vi "SwitchFinder.vi"(10 "All Lines in":T1) -> (2 "All Lines out":T1)   [LabVIEW 2014]
uses:
  Libraries/Map Data Folder/All-Lines.ctl
  Libraries/Map Data Folder/LineCluster.ctl
  Libraries/Map Data Folder/LineConnection.ctl
  Libraries/Map Data Folder/Map Data.lvlib
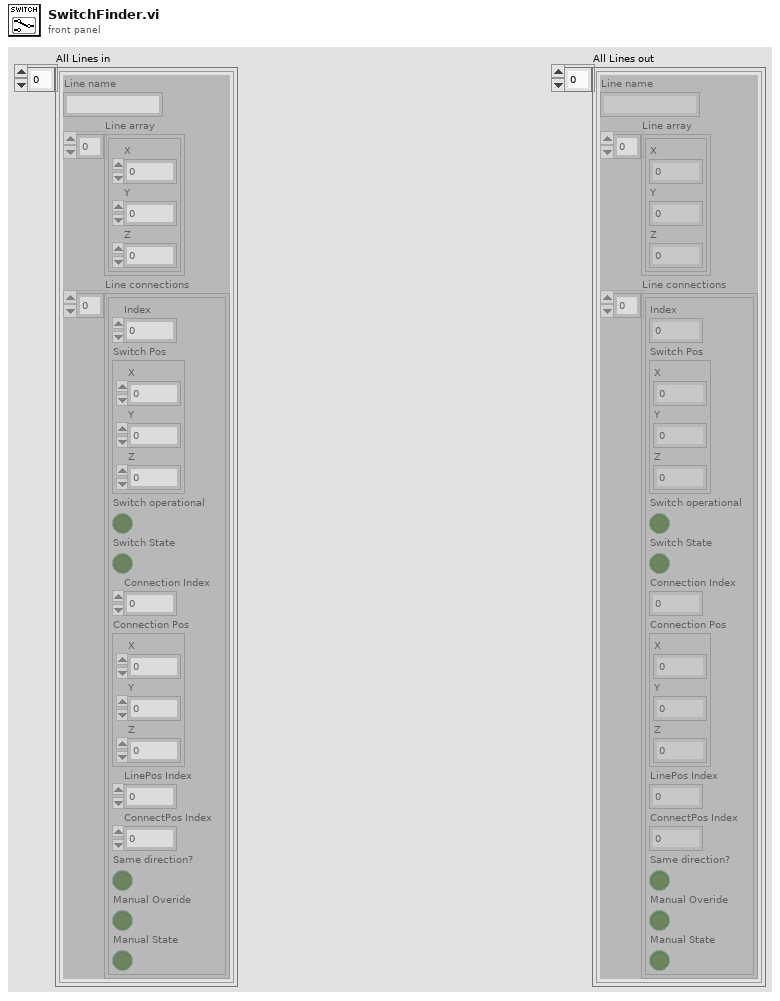
[diagram p1: front panel]
types:
  T1 = typedef "Map Data.lvlib/All-Lines.ctl" = T2[]
  T2 = typedef "Map Data.lvlib/LineCluster.ctl" = cluster{"Line name":string, "Line array":cluster{"X":dbl, "Y":dbl, "Z":dbl}[], "Line connections":T3[]}
  T3 = typedef "LineConnection.ctl" = cluster{"Index":i32, "Switch Pos":cluster{"X":dbl, "Y":dbl, "Z":dbl}, "Switch operational":bool, "Switch State":bool, "Connection Index":i32, "Connection Pos":cluster{"X":dbl, "Y":dbl, "Z":dbl}, "LinePos Index":i32, "ConnectPos Index":i32, "Same direction?":bool, "Manual Overide":bool, "Manual State":bool}
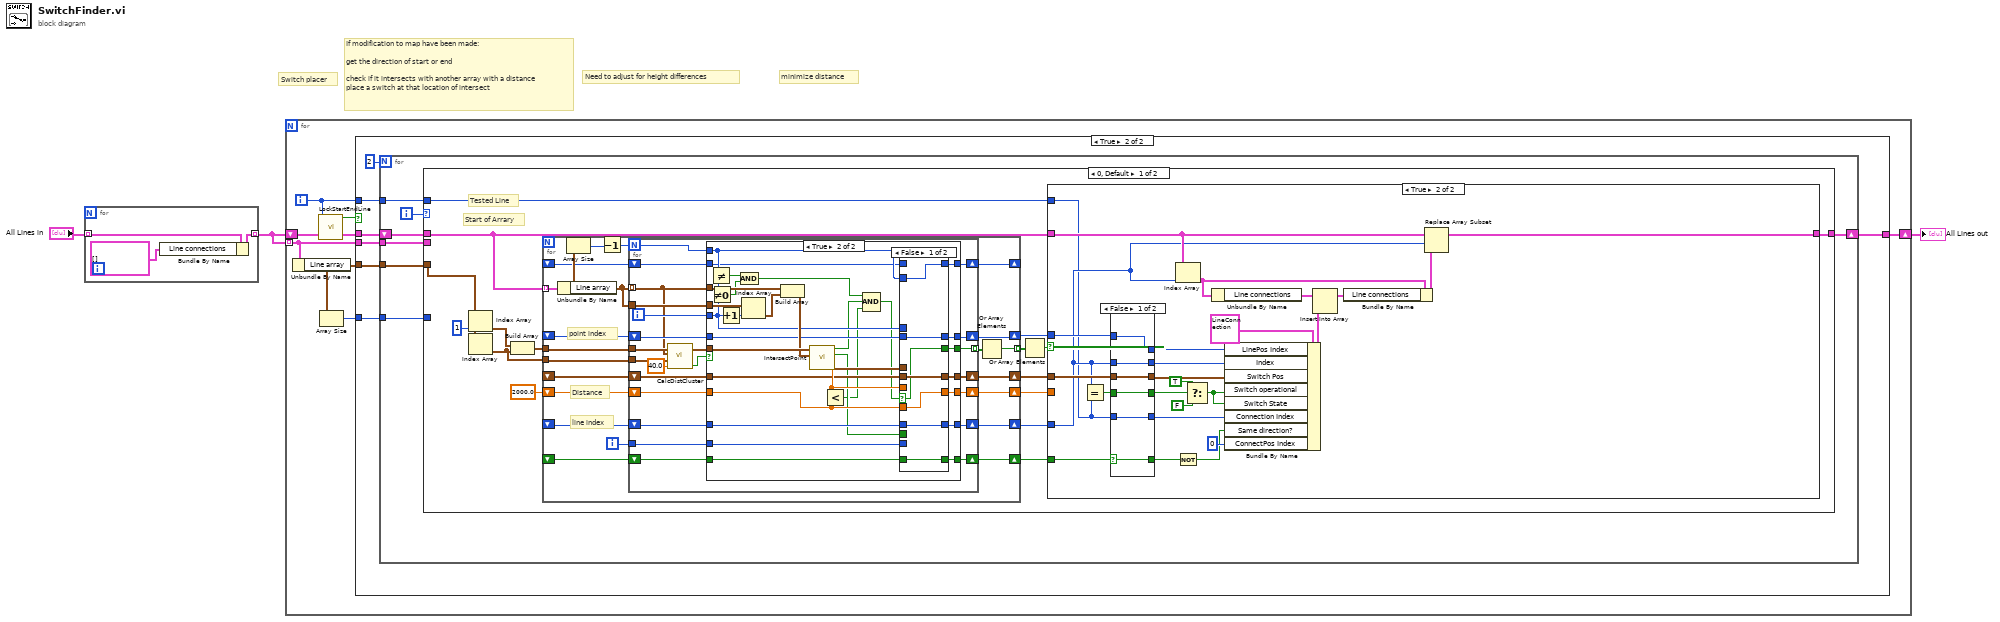
[diagram p0: block diagram]
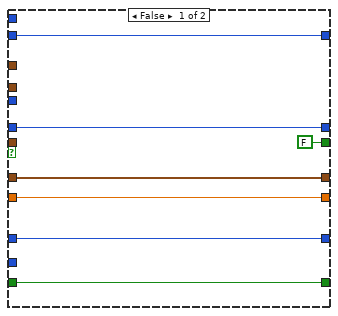
[diagram p5: hidden frame]
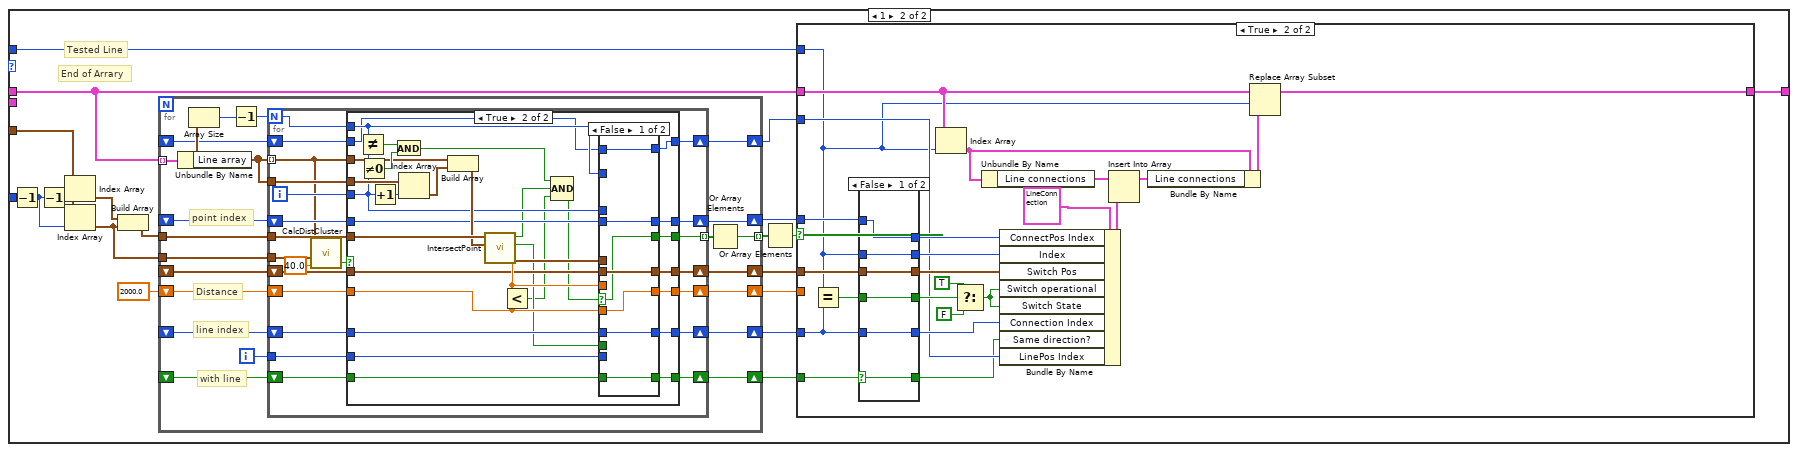
[diagram p7: hidden frame]
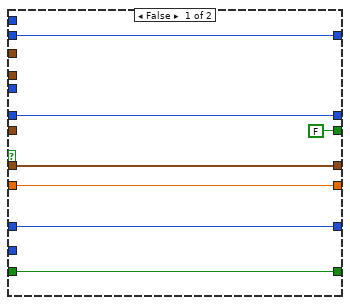
[diagram p10: hidden frame]
diagram:
  # "minimize distance"
  # "Need to adjust for height differences"
  # "If modification to map have been made:\n\nget the direction of start or end\n\ncheck if it intersects with another array with a distance\nplace a switch at that location of intersect"
  # "Switch placer"
  n1 = for {
    tunnel: [w5] -> w2 mode=indexing
    tunnel: "All Lines in" -> [w6] mode=indexing
    n2 = Bundle By Name(cluster=w6, "Line connections"=T3[] []) -> (w5:T2)
  }
  n3 = for {
    tunnel: w2 -> [w10] mode=indexing
    shift-right: [w7] -> w3
    shift-left: w2 -> [w9]
    i -> [w8]
    n4 = Unbundle By Name(w10) -> ("Line array"=w12:cluster{"X":dbl, "Y":dbl, "Z":dbl}[])
    n5 = call "LockStartEndLine.vi"("index"=w8, "All Lines"=w9) -> ("Not Locked?"=w11:bool)  [unwired: 9 in]
    n6 = Array Size(array=w12) -> (size(s)=w13:i32)
    n7 = case shown="True" w11 {
      tunnel: w13 -> [_ w21]
      tunnel: w12 -> [_ w20]
      tunnel: w10 -> [_ w16]
      tunnel: w9 -> [w14 w18]
      tunnel: w8 -> [_ w17]
      tunnel: [w14 w15] -> w7
      frame False {
      }
      frame True {
        n8 = for {
          N: 2 -> [_]
          tunnel: w21 -> [w28]
          tunnel: w20 -> [w27]
          shift-right: [w24] -> w15
          shift-left: w18 -> [w25]
          tunnel: w17 -> [w23]
          tunnel: w16 -> [w22]
          i -> [w26]
          n9 = case shown="0, Default" w26 {
            tunnel: w28 -> [_ w183]
            tunnel: w27 -> [w42 w194]
            tunnel: w25 -> [w37 w190]
            tunnel: [w38 w191] -> w24
            tunnel: w23 -> [w36 w189]
            tunnel: w22 -> [_ _]
            frame 0, Default {
              # "Tested Line"
              # "Start of Arrary"
              n10 = Index Array(array=w42, index=1) -> (element=w44:cluster{"X":dbl, "Y":dbl, "Z":dbl})
              n11 = Index Array(array=w42) -> (element=w30:cluster{"X":dbl, "Y":dbl, "Z":dbl})  [unwired: 1 in]
              n12 = Build Array(w44, w30) -> (w43:cluster{"X":dbl, "Y":dbl, "Z":dbl}[])
              n13 = for {
                tunnel: w43 -> [w103]
                tunnel: w37 -> [w102] mode=indexing
                shift-right: [w99] -> w32
                shift-left: 2000.0 ("Distance") -> [w98]
                shift-right: [w96] -> w34
                shift-left: _ -> [w95]
                shift-right: [w92] -> w31
                shift-left: _ -> [w93]
                tunnel: [w90] -> w40 mode=indexing
                shift-right: [w89] -> w33
                shift-left: _ -> [w88]
                tunnel: w30 -> [w87]
                shift-right: [w86] -> w29
                shift-left: _ -> [w85]
                shift-right: [w84] -> _
                shift-left: _ -> [w83]
                i -> [w91]
                # "Distance"
                # "line index"
                # "point index"
                n14 = Unbundle By Name(w102) -> ("Line array"=w101:cluster{"X":dbl, "Y":dbl, "Z":dbl}[])
                n15 = Array Size(array=w101) -> (size(s)=w94:i32)
                n16 = Decrement(x=w94) -> (x-1=w100:i32)
                n17 = for {
                  N: w100 -> [w117]
                  tunnel: w103 -> [w125]
                  tunnel: w101 -> [w109] mode=indexing
                  tunnel: w101 -> [w124]
                  tunnel: [w120] -> w97 mode=indexing
                  shift-right: [w122] -> w99
                  shift-left: w98 -> [w123]
                  shift-right: [w121] -> w96
                  shift-left: w95 -> [w119]
                  tunnel: w91 -> [w115]
                  shift-right: [w116] -> w92
                  shift-left: w93 -> [w114]
                  shift-right: [w113] -> w89
                  shift-left: w88 -> [w112]
                  tunnel: w87 -> [w108]
                  shift-right: [w107] -> w86
                  shift-left: w85 -> [w106]
                  shift-right: [w105] -> w84
                  shift-left: w83 -> [w104]
                  i -> [w118]
                  n18 = call "CalcDistCluster.vi"("Less than"=40.0, "element 2"=w108, "element"=w109) -> ("Less than?"=w110:bool)  [unwired: 7 in, 1 out]
                  n19 = case shown="True" w110 {
                    tunnel: w125 -> [_ w163]
                    tunnel: w124 -> [_ w162]
                    tunnel: w109 -> [_ w160]
                    tunnel: w123 -> [w129 w157]
                    tunnel: [w129 w155] -> w122
                    tunnel: [w132 w154] -> w121
                    tunnel: [FALSE w153] -> w120
                    tunnel: w119 -> [w132 w152]
                    tunnel: w118 -> [_ w151]
                    tunnel: w117 -> [_ w139]
                    tunnel: [w128 w148] -> w116
                    tunnel: w115 -> [_ w147]
                    tunnel: w114 -> [w128 w146]
                    tunnel: [w130 w144] -> w113
                    tunnel: w112 -> [w130 w143]
                    tunnel: [w127 w141] -> w107
                    tunnel: w106 -> [w127 w140]
                    tunnel: [w126 w138] -> w105
                    tunnel: w104 -> [w126 w137]
                    frame False {
                    }
                    frame True {
                      n20 = Not Equal?(x=w139, y=w151) -> (x != y?=w150:bool)
                      n21 = Not Equal To 0?(x=w151) -> (x != 0?=w149:bool)
                      n22 = Increment(x=w151) -> (x+1=w161:i32)
                      n23 = And(x=w150, y=w149) -> (x .and. y?=w136:bool)
                      n24 = Index Array(array=w162, index=w161) -> (element=w159:cluster{"X":dbl, "Y":dbl, "Z":dbl})
                      n25 = Build Array(w160, w159) -> (w158:cluster{"X":dbl, "Y":dbl, "Z":dbl}[])
                      n26 = call "IntersectPoint.vi"("Against Array"=w158, "Test Array"=w163) -> ("Intersect Point"=w145:cluster{"X":dbl, "Y":dbl, "Z":dbl}, "Distance"=w156:dbl, "With Line?"=w142:bool, "Check"=w135:bool)  [unwired: 6 in]
                      n27 = Less?(x=w156, y=w157) -> (x < y?=w134:bool)
                      n28 = Compound Arithmetic op=AND(w136, w135, w134) -> (w133:bool)
                      n29 = case shown="False" w133 {
                        selector: w133 -> [w164 w171]
                        tunnel: w157 -> [w170 _]
                        tunnel: w156 -> [_ w177]
                        tunnel: [w170 w177] -> w155
                        tunnel: w152 -> [w169 _]
                        tunnel: [w169 w176] -> w154
                        tunnel: [w164 w171] -> w153
                        tunnel: w151 -> [_ w176]
                        tunnel: [w168 w175] -> w148
                        tunnel: w147 -> [_ w175]
                        tunnel: w146 -> [w168 _]
                        tunnel: w145 -> [_ w174]
                        tunnel: [w167 w174] -> w144
                        tunnel: w143 -> [w167 _]
                        tunnel: w142 -> [_ w173]
                        tunnel: [w166 w173] -> w141
                        tunnel: w140 -> [w166 _]
                        tunnel: w139 -> [w165 _]
                        tunnel: [w165 w172] -> w138
                        tunnel: w137 -> [_ w172]
                        frame False {
                        }
                        frame True {
                        }
                      }
                    }
                  }
                }
                n30 = Or Array Elements(Boolean array=w97) -> (logical OR=w90:bool)
              }
              n31 = Or Array Elements(Boolean array=w40) -> (logical OR=w35:bool)
              n32 = case shown="True" w35 {
                tunnel: [w45 w50] -> w38
                tunnel: w37 -> [w45 w66]
                tunnel: w36 -> [_ w48]
                tunnel: w34 -> [_ w56]
                tunnel: w33 -> [_ w64]
                tunnel: w32 -> [_ _]
                tunnel: w31 -> [_ w49]
                tunnel: w29 -> [_ w65]
                frame False {
                }
                frame True {
                  n33 = Equal?(x=w49, y=w48) -> (x = y?=w58:bool)
                  n34 = case shown="False" w65 {
                    selector: w65 -> [w71 w78]
                    tunnel: w48 -> [w75 w82]
                    tunnel: [w75 w82] -> w62
                    tunnel: [w76 w81] -> w51
                    tunnel: w64 -> [w76 w81]
                    tunnel: w49 -> [w74 w77]
                    tunnel: [w74 w77] -> w63
                    tunnel: w58 -> [w73 w80]
                    tunnel: [w73 w80] -> w57
                    tunnel: w56 -> [w72 w79]
                    tunnel: [w72 w79] -> w53
                    tunnel: [w71 w78] -> w54
                    frame False {
                    }
                    frame True {
                    }
                  }
                  n35 = Index Array(array=w66, index=w49) -> (element=w70:T2)
                  n36 = Not(x=w54) -> (.not. x?=w47:bool)
                  n37 = Select(t=TRUE ("Switch operational"), s=w57, f=FALSE ("Switch operational")) -> (s? t:f=w61:bool)
                  n38 = Unbundle By Name(w70) -> ("Line connections"=w67:T3[])
                  n39 = Bundle By Name(cluster=T3 {"Index"=0, "Switch Pos"={"X"=0.0, "Y"=0.0, "Z"=0.0}, "Switch operational"=FALSE, "Switch State"=FALSE, "Connection Index"=0, "Connection Pos"={"X"=0.0, "Y"=0.0, "Z"=0.0}, "LinePos Index"=0, "ConnectPos Index"=0, "Same direction?"=FALSE, "Manual Overide"=FALSE, "Manual State"=FALSE}, "LinePos Index"=w53, "Index"=w63, "Switch Pos"=w51, "Switch operational"=w61, "Switch State"=w61, "Connection Index"=w62, "Same direction?"=w47, "ConnectPos Index"=0) -> (w55:T3)
                  n40 = Insert Into Array(array=w67, new element=w55) -> (w69:T3[])  [unwired: 1 in]
                  n41 = Bundle By Name(cluster=w70, "Line connections"=w69) -> (w68:T2)
                  n42 = Replace Array Subset(array=w66, new element=w68, index=w49) -> (w50:T2[])
                }
              }
            }
            frame 1 {
              # "Tested Line"
              # "End of Arrary"
              n43 = Decrement(x=w183) -> (x-1=w182:i32)
              n44 = Decrement(x=w182) -> (x-1=w181:i32)
              n45 = Index Array(array=w194, index=w181) -> (element=w196:cluster{"X":dbl, "Y":dbl, "Z":dbl})
              n46 = Index Array(array=w194, index=w182) -> (element=w180:cluster{"X":dbl, "Y":dbl, "Z":dbl})
              n47 = Build Array(w196, w180) -> (w195:cluster{"X":dbl, "Y":dbl, "Z":dbl}[])
              n48 = for {
                tunnel: w195 -> [w254]
                tunnel: w190 -> [w253] mode=indexing
                shift-right: [w250] -> w185
                shift-left: 2000.0 ("Distance") -> [w249]
                shift-right: [w247] -> w187
                shift-left: _ -> [w246]
                shift-right: [w243] -> w184
                shift-left: _ -> [w244]
                tunnel: [w241] -> w192 mode=indexing
                shift-right: [w240] -> w186
                shift-left: _ -> [w239]
                tunnel: w180 -> [w238]
                shift-right: [w237] -> w179
                shift-left: _ -> [w236]
                shift-right: [w235] -> w178
                shift-left: _ -> [w234]
                i -> [w242]
                # "with line"
                # "Distance"
                # "line index"
                # "point index"
                n49 = Unbundle By Name(w253) -> ("Line array"=w252:cluster{"X":dbl, "Y":dbl, "Z":dbl}[])
                n50 = Array Size(array=w252) -> (size(s)=w245:i32)
                n51 = Decrement(x=w245) -> (x-1=w251:i32)
                n52 = for {
                  N: w251 -> [w257]
                  tunnel: w254 -> [w276]
                  tunnel: w252 -> [w263] mode=indexing
                  tunnel: w252 -> [w275]
                  tunnel: [w271] -> w248 mode=indexing
                  shift-right: [w273] -> w250
                  shift-left: w249 -> [w274]
                  shift-right: [w272] -> w247
                  shift-left: w246 -> [w270]
                  tunnel: w242 -> [w267]
                  shift-right: [w268] -> w243
                  shift-left: w244 -> [w266]
                  shift-right: [w265] -> w240
                  shift-left: w239 -> [w264]
                  tunnel: w238 -> [w262]
                  shift-right: [w259] -> w237
                  shift-left: w236 -> [w258]
                  shift-right: [w256] -> w235
                  shift-left: w234 -> [w255]
                  i -> [w269]
                  n53 = call "CalcDistCluster.vi"("Less than"=40.0, "element 2"=w262, "element"=w263) -> ("Less than?"=w260:bool)  [unwired: 7 in, 1 out]
                  n54 = case shown="True" w260 {
                    tunnel: w276 -> [_ w314]
                    tunnel: w275 -> [_ w313]
                    tunnel: w274 -> [w280 w309]
                    tunnel: [w280 w307] -> w273
                    tunnel: [w283 w306] -> w272
                    tunnel: [FALSE w305] -> w271
                    tunnel: w270 -> [w283 w304]
                    tunnel: w269 -> [_ w303]
                    tunnel: [w281 w300] -> w268
                    tunnel: w267 -> [_ w299]
                    tunnel: w266 -> [w281 w298]
                    tunnel: [w282 w296] -> w265
                    tunnel: w264 -> [w282 w295]
                    tunnel: w263 -> [_ w294]
                    tunnel: [w278 w292] -> w259
                    tunnel: w258 -> [w278 w291]
                    tunnel: w257 -> [_ w290]
                    tunnel: [w277 w288] -> w256
                    tunnel: w255 -> [w277 w289]
                    frame False {
                    }
                    frame True {
                      n55 = Not Equal?(x=w290, y=w303) -> (x != y?=w302:bool)
                      n56 = Not Equal To 0?(x=w303) -> (x != 0?=w301:bool)
                      n57 = Increment(x=w303) -> (x+1=w312:i32)
                      n58 = And(x=w302, y=w301) -> (x .and. y?=w285:bool)
                      n59 = Index Array(array=w313, index=w312) -> (element=w311:cluster{"X":dbl, "Y":dbl, "Z":dbl})
                      n60 = Build Array(w294, w311) -> (w310:cluster{"X":dbl, "Y":dbl, "Z":dbl}[])
                      n61 = call "IntersectPoint.vi"("Against Array"=w310, "Test Array"=w314) -> ("Intersect Point"=w297:cluster{"X":dbl, "Y":dbl, "Z":dbl}, "Distance"=w308:dbl, "With Line?"=w293:bool, "Check"=w286:bool)  [unwired: 6 in]
                      n62 = Less?(x=w308, y=w309) -> (x < y?=w287:bool)
                      n63 = Compound Arithmetic op=AND(w285, w286, w287) -> (w284:bool)
                      n64 = case shown="False" w284 {
                        selector: w284 -> [w315 w322]
                        tunnel: w309 -> [w321 _]
                        tunnel: w308 -> [_ w328]
                        tunnel: [w321 w328] -> w307
                        tunnel: w304 -> [w320 _]
                        tunnel: [w320 w327] -> w306
                        tunnel: [w315 w322] -> w305
                        tunnel: w303 -> [_ w327]
                        tunnel: [w319 w326] -> w300
                        tunnel: w299 -> [_ w326]
                        tunnel: w298 -> [w319 _]
                        tunnel: w297 -> [_ w325]
                        tunnel: [w318 w325] -> w296
                        tunnel: w295 -> [w318 _]
                        tunnel: w293 -> [_ w324]
                        tunnel: [w317 w324] -> w292
                        tunnel: w291 -> [w317 _]
                        tunnel: w290 -> [_ w323]
                        tunnel: w289 -> [w316 _]
                        tunnel: [w316 w323] -> w288
                        frame False {
                        }
                        frame True {
                        }
                      }
                    }
                  }
                }
                n65 = Or Array Elements(Boolean array=w248) -> (logical OR=w241:bool)
              }
              n66 = Or Array Elements(Boolean array=w192) -> (logical OR=w188:bool)
              n67 = case shown="True" w188 {
                tunnel: [w197 w202] -> w191
                tunnel: w190 -> [w197 w216]
                tunnel: w189 -> [_ w200]
                tunnel: w187 -> [_ w207]
                tunnel: w186 -> [_ w214]
                tunnel: w185 -> [_ _]
                tunnel: w184 -> [_ w201]
                tunnel: w179 -> [_ w215]
                tunnel: w178 -> [_ w203]
                frame False {
                }
                frame True {
                  n68 = Equal?(x=w200, y=w201) -> (x = y?=w209:bool)
                  n69 = case shown="False" w215 {
                    selector: w215 -> [w223 w228]
                    tunnel: w201 -> [w222 w231]
                    tunnel: [w222 w231] -> w206
                    tunnel: w200 -> [w227 w232]
                    tunnel: [w227 w232] -> w213
                    tunnel: w214 -> [w226 w233]
                    tunnel: [w226 w233] -> w204
                    tunnel: w209 -> [w225 w230]
                    tunnel: [w225 w230] -> w208
                    tunnel: w207 -> [w224 w229]
                    tunnel: [w224 w229] -> w205
                    tunnel: [w223 w228] -> w199
                    frame False {
                    }
                    frame True {
                    }
                  }
                  n70 = Index Array(array=w216, index=w200) -> (element=w220:T2)
                  n71 = Select(t=TRUE, s=w208, f=FALSE ("Switch State")) -> (s? t:f=w210:bool)
                  n72 = Unbundle By Name(w220) -> ("Line connections"=w217:T3[])
                  n73 = Bundle By Name(cluster=T3 {"Index"=0, "Switch Pos"={"X"=0.0, "Y"=0.0, "Z"=0.0}, "Switch operational"=FALSE, "Switch State"=FALSE, "Connection Index"=0, "Connection Pos"={"X"=0.0, "Y"=0.0, "Z"=0.0}, "LinePos Index"=0, "ConnectPos Index"=0, "Same direction?"=FALSE, "Manual Overide"=FALSE, "Manual State"=FALSE}, "ConnectPos Index"=w205, "Index"=w213, "Switch Pos"=w204, "Switch operational"=w210, "Switch State"=w210, "Connection Index"=w206, "Same direction?"=w199, "LinePos Index"=w203) -> (w221:T3)
                  n74 = Insert Into Array(array=w217, new element=w221) -> (w219:T3[])  [unwired: 1 in]
                  n75 = Bundle By Name(cluster=w220, "Line connections"=w219) -> (w218:T2)
                  n76 = Replace Array Subset(array=w216, new element=w218, index=w200) -> (w202:T2[])
                }
              }
            }
          }
        }
      }
    }
  }
  "All Lines out" <- w3
